vi "DivBinning.vi"(7 "Settings.number of cam":dbl, 10 "offset":dbl, 11 "spec cluster 3":cluster{"dp [MeV/C]":dbl[], dbl[]}[](graph)) -> (1 "spec cluster":cluster{"dp [MeV/C]":dbl[], dbl[]}(graph), 2 "divergence":waveform(dbl), 5 "time:div":u32)   [LabVIEW 2020]
panel:
  out "Numeric":dbl
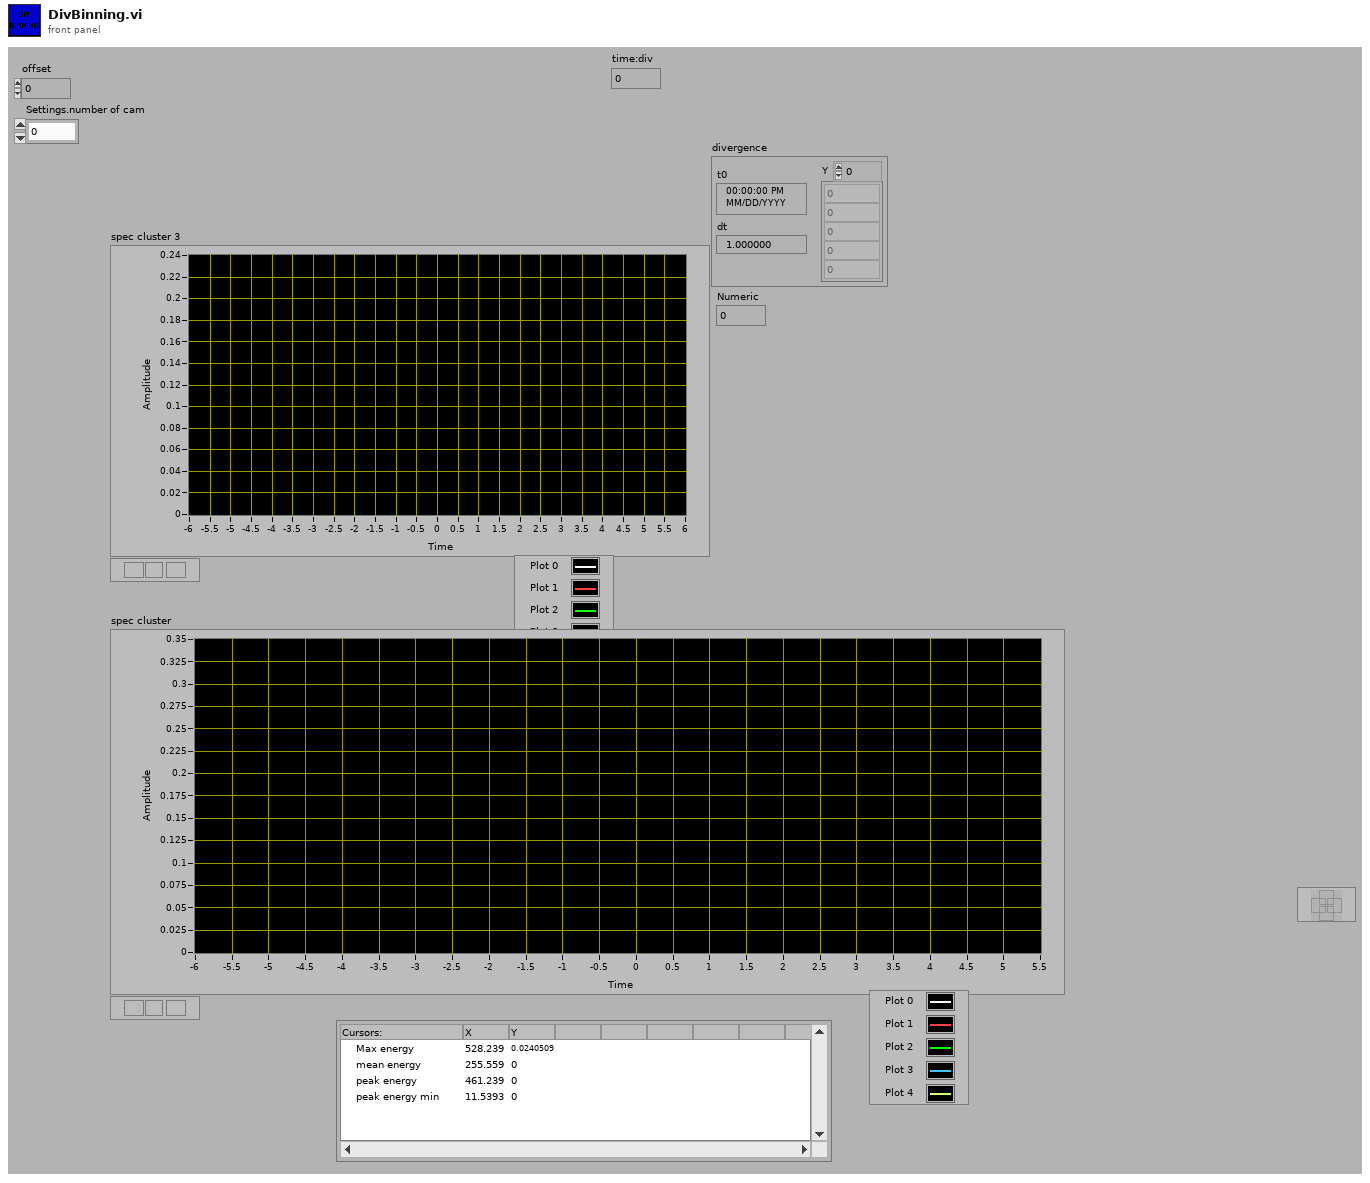
[diagram p1: front panel]
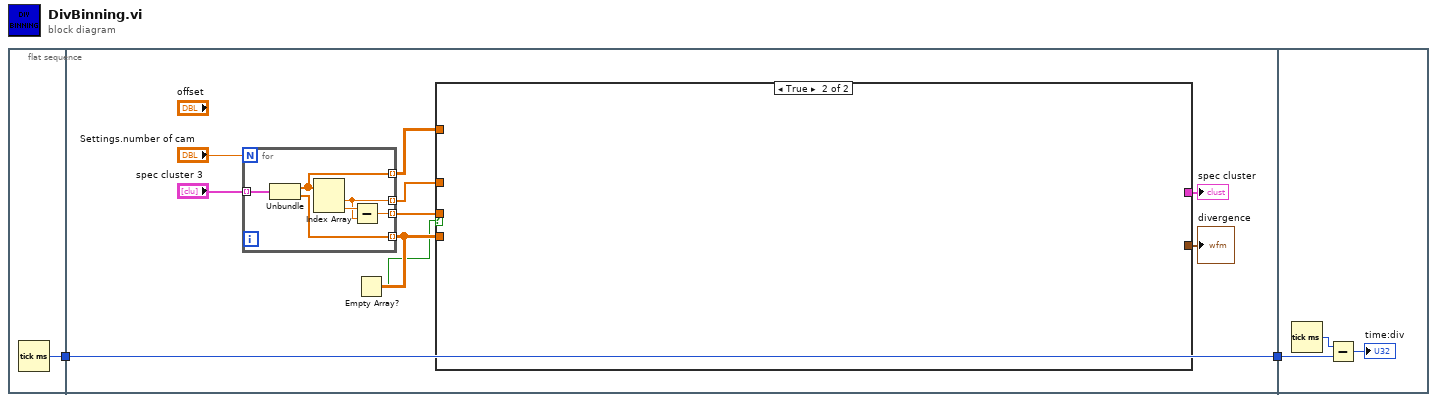
[diagram p0: block diagram]
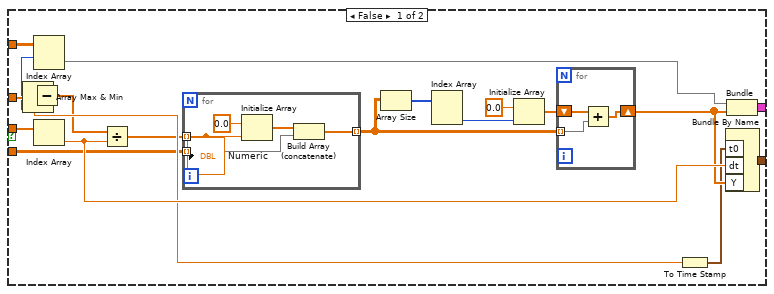
[diagram p2: hidden frame]
diagram:
  n1 = flat-sequence {
    tunnel: [w3] -> w2
    tunnel: w2 -> [w12]
    tunnel: [w12] -> w1
    tunnel: w1 -> [w48]
    frame #0 {
      n2 = Tick Count (ms)() -> (millisecond timer value=w3:u32)
    }
    frame #1 {
      n3 = for {
        N: "Settings.number of cam" -> [_]
        tunnel: "spec cluster 3" -> [w46] mode=indexing
        tunnel: [w44] -> w8 mode=indexing
        tunnel: [w43] -> w7 mode=indexing
        tunnel: [w42] -> w5 mode=indexing
        tunnel: [w41] -> w6 mode=indexing
        n4 = Unbundle(w46) -> ("dp [MeV/C]"=w41:dbl[], w42:dbl[])
        n5 = Index Array(array=w41) -> (element #1=w44:dbl, element #2=w45:dbl)  [unwired: 2 in]
        n6 = Subtract(x=w45, y=w44) -> (x-y=w43:dbl)
      }
      n7 = Empty Array?(array=w5) -> (empty?=w4:bool)
      n8 = case shown="True" w4 {
        tunnel: [w28 _] -> w10
        tunnel: [w27 _] -> w9
        tunnel: w8 -> [w25 _]
        tunnel: w7 -> [w24 _]
        tunnel: w6 -> [w16 _]
        tunnel: w5 -> [w14 _]
        frame False {
          n9 = Array Max & Min(array=w25) -> (min value=w26:dbl, min index (indices)=w15:i32)  [unwired: 2 out]
          n10 = Subtract(x=w25, y=w26) -> (x-y=w23:dbl[])
          n11 = Index Array(array=w16, index (row)=w15) -> (element=w31:dbl[])  [unwired: 1 in]
          n12 = Index Array(array=w24) -> (element=w32:dbl)  [unwired: 1 in]
          n13 = Divide(x=w23, y=w32) -> (x/y=w22:dbl[])
          n14 = for {
            tunnel: w22 -> [w40] mode=indexing
            tunnel: w14 -> [w38] mode=indexing
            tunnel: [w36] -> w18 mode=indexing
            n15 = Initialize Array(0.0 ("element"), w40) -> (w37:dbl[])
            n16 = Build Array (concatenate)(w37, w38) -> (w36:dbl[])
            "Numeric" <- w40
          }
          n17 = Array Size(array=w18) -> (size(s)=w21:i32[])
          n18 = Index Array(array=w21) -> (element #2=w20:i32)  [unwired: 2 in, 1 out]
          n19 = Initialize Array(0.0 ("element"), w20) -> (w17:dbl[])
          n20 = for {
            tunnel: w18 -> [w34] mode=indexing
            shift-right: [w33] -> w30
            shift-left: w17 -> [w35]
            n21 = Add(x=w35, y=w34) -> (x+y=w33:dbl[])
          }
          n22 = To Time Stamp(1:w26) -> (0:w29:timestamp)
          n23 = Bundle By Name("t0"=w29, "dt"=w32, "Y"=w30) -> (w28:waveform(dbl))  [unwired: 1 in]
          n24 = Bundle("dp [MeV/C]"=w31, w30) -> (w27:cluster{"dp [MeV/C]":dbl[], dbl[]})  [unwired: 1 in]
        }
        frame True {
        }
      }
      "spec cluster" <- w9
      "divergence" <- w10
    }
    frame #2 {
      n25 = Tick Count (ms)() -> (millisecond timer value=w49:u32)
      n26 = Subtract(x=w49, y=w48) -> (x-y=→"time:div":u32)
    }
  }
